vi "Configure RF Input.vi"(0 "VISA resource name":refnum<visa-resource-name>, 1 "Preselector Frequency (0 MHz)":dbl format="%^#_6g", 5 "Maximum RF Attenuation (0 dB)":dbl, 7 "Minimum RF Attenuation (0 dB)":dbl, 9 "RF Attenuation (0 dB)":dbl format="%^#_6g", 11 "error in (no error)":errorcluster, 12 "RF Input Port Coupling (AC)":i32(ring) items=["AC", "DC"]) -> (4 "VISA resource name out":refnum<visa-resource-name>, 15 "error out":errorcluster)   [LabVIEW 2014, in "Agilent ESA PSA Series.lvlib"]
doc: "Configures the input options of the Noise Figure personality.\n\n<B>Note:</B> \n\nThis VI is only valid in Noise Figure personality. Use <B>Switch Personality</B> VI to switch to Noise Figure before calling this VI."
uses:
  Agilent ESA PSA Series.lvlib
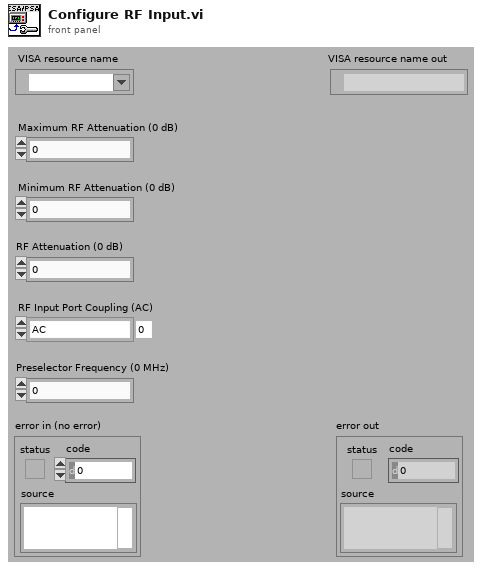
[diagram p1: front panel]
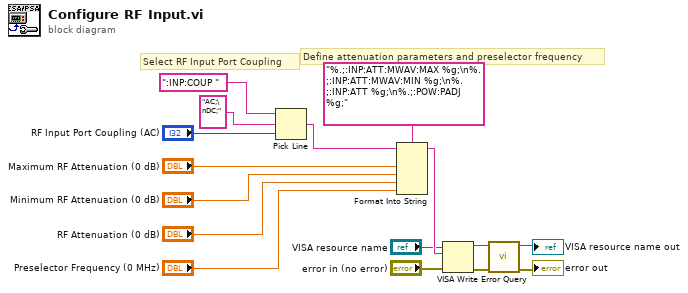
[diagram p0: block diagram]
diagram:
  # "Define attenuation parameters and preselector frequency"
  # "Select RF Input Port Coupling"
  n1 = Pick Line(string ("")=":INP:COUP ", multi-line string="AC;\nDC;", line index="RF Input Port Coupling (AC)") -> (output string=w7:string)
  n2 = Format Into String(format string="%.;:INP:ATT:MWAV:MAX %g;\n%.;:INP:ATT:MWAV:MIN %g;\n%.;:INP:ATT %g;\n%.;:POW:PADJ %g;", initial string=w7, "Maximum RF Attenuation (0 dB)", "Minimum RF Attenuation (0 dB)", "RF Attenuation (0 dB)", "Preselector Frequency (0 MHz)") -> (resulting string=w3:string)  [unwired: 1 in, 1 out]
  n3 = VISA Write(VISA resource name="VISA resource name", write buffer=w3, error in (no error)="error in (no error)") -> (VISA resource name out=w14:refnum<visa-resource-name>, error out=w13:errorcluster)  [unwired: 1 out]
  n4 = call "Error Query.vi"("error in (no error)"=w13, "VISA resource name"=w14) -> ("error out"=→"error out":errorcluster, "VISA resource name out"=→"VISA resource name out":refnum<visa-resource-name>)  [unwired: 6 in, 2 out]
